vi "MM_WireControlsToBundler.vi"(7 "MessageClassRef":refnum<vi>, 8 "error in (no error)":errorcluster, 10 "Controls":refnum<vi>[](array[refnum]), 11 "vi reference in":refnum<vi>) -> (0 "error out":errorcluster, 3 "vi reference out":refnum<vi>)   [LabVIEW 2014]
uses:
  <vilib>/Utility/traverseref.llb/TRef TravTarget.ctl
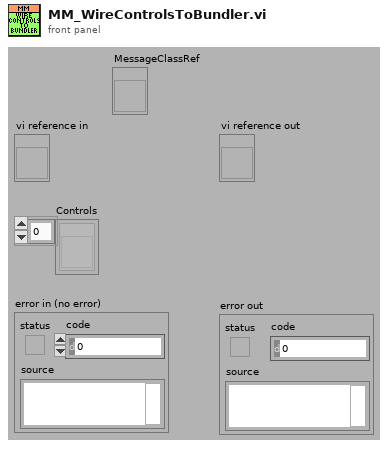
[diagram p1: front panel]
types:
  T1 = typedef "TRef TravTarget.ctl" = enum16{"FP", "BD", "Other"}
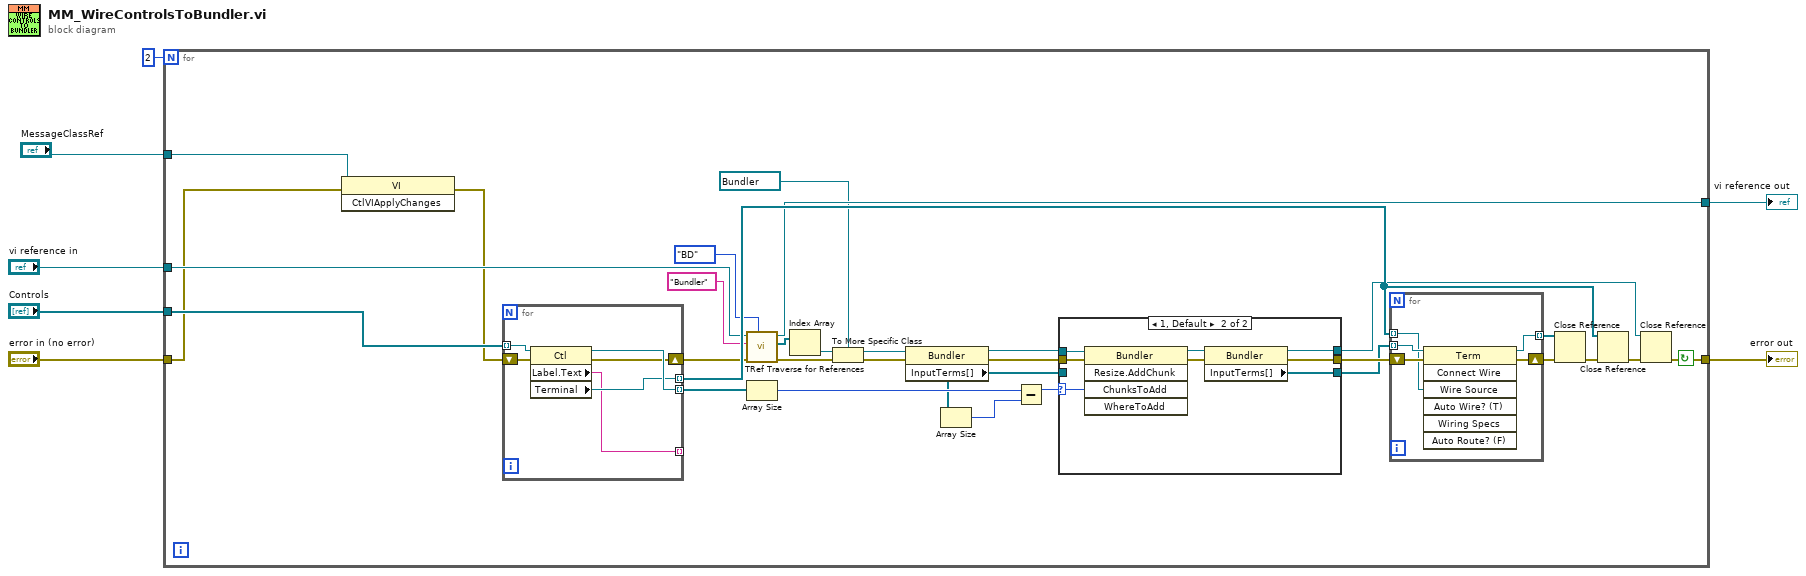
[diagram p0: block diagram]
diagram:
  n1 = for {
    N: 2 -> [_]
    tunnel: [w10] -> w7
    tunnel: [w35] -> w6
    tunnel: "Controls" -> [w30]
    tunnel: "vi reference in" -> [w29]
    tunnel: "MessageClassRef" -> [w9]
    tunnel: "error in (no error)" -> [w8]
    stop <- w10 continue-if-true
    n2 = invoke class="VI" method="CtlVIApplyChanges"(reference=w9, error in=w8) -> (error out=w11:errorcluster)  [unwired: 1 in, 2 out]
    n3 = for {
      tunnel: [w55] -> _ mode=indexing
      tunnel: [w60] -> w32 mode=indexing
      tunnel: w30 -> [w59] mode=indexing
      shift-right: [w57] -> w31
      shift-left: w11 -> [w58]
      tunnel: [w56] -> w37 mode=indexing
      n4 = property class="Ctl"(reference=w59, error in=w58) -> (reference out=w60:refnum<vi>, error out=w57:errorcluster, "Label.Text"=w55:string, "Terminal"=w56:refnum<vi>)
    }
    n5 = call <vilib>:"TRef Traverse for References.vi"("Traverse Target"=TRef_TravTarget."BD", "error in (no error)"=w31, "Class Name"="Bundler", "VI Refnum"=w29) -> ("error out"=w28:errorcluster, "References"=w26:refnum<vi>[], "dup VI Refnum"=w35:refnum<vi>)  [unwired: 4 in, 1 out]
    n6 = Array Size(array=w32) -> (size(s)=w18:i32)
    n7 = Index Array(array=w26) -> (element=w27:refnum<vi>)  [unwired: 1 in]
    n8 = To More Specific Class(target class=refnum<vi> refnum ("reference"), reference=w27, error in=w28) -> (specific class reference=w22:refnum<vi>, error out=w21:errorcluster)
    n9 = property class="Bundler"(reference=w22, error in=w21) -> (reference out=w20:refnum<vi>, error out=w19:errorcluster, "InputTerms[]"=w15:refnum<vi>[])
    n10 = Array Size(array=w15) -> (size(s)=w17:i32)
    n11 = Subtract(x=w18, y=w17) -> (x-y=w16:i32)
    n12 = case shown="1, Default" w16 {
      selector: w16 -> [_ w47]
      tunnel: [w40 w43] -> w14
      tunnel: [w41 w44] -> w13
      tunnel: w19 -> [w40 w49]
      tunnel: w20 -> [w41 w48]
      tunnel: w15 -> [w39 _]
      tunnel: [w39 w42] -> w12
      frame ..0 {
      }
      frame 1, Default {
        n13 = invoke class="Bundler" method="Resize.AddChunk"(reference=w48, error in=w49, "ChunksToAdd"=w47) -> (reference out=w46:refnum<vi>, error out=w45:errorcluster)  [unwired: 2 in, 3 out]
        n14 = property class="Bundler"(reference=w46, error in=w45) -> (reference out=w44:refnum<vi>, error out=w43:errorcluster, "InputTerms[]"=w42:refnum<vi>[])
      }
    }
    n15 = for {
      tunnel: w37 -> [w52] mode=indexing
      shift-right: [w51] -> w33
      shift-left: w14 -> [w53]
      tunnel: w12 -> [w54] mode=indexing
      tunnel: [w50] -> w34 mode=indexing
      n16 = invoke class="Term" method="Connect Wire"(reference=w54, error in=w53, "Wire Source"=w52) -> (reference out=w50:refnum<vi>, error out=w51:errorcluster)  [unwired: 4 in, 5 out]
    }
    n17 = Close Reference(reference=w34, error in (no error)=w33) -> (error out=w36:errorcluster)
    n18 = Close Reference(reference=w37, error in (no error)=w36) -> (error out=w38:errorcluster)
    n19 = Close Reference(reference=w13, error in (no error)=w38) -> (error out=w10:errorcluster)
  }
  "error out" <- w7
  "vi reference out" <- w6
